vi "WriteBarcodeType.vi"(4 "error in (no error)":errorcluster, 5 "Value":T2, 6 "Container State":T3, 7 "Display State In":T1) -> (0 "error out":errorcluster, 3 "Display State Out":T1)   [LabVIEW 2013, in "BarCodes.lvlib" / "Barcode.xctl"]
uses:
  Barcode.xctl
  <vilib>/_xctls/Container State.ctl
  BarcodeType.ctl
  State.ctl
  <vilib>/_xctls/XControlSupport.lvlib
  BarCodes.lvlib
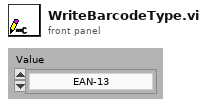
[diagram p1: front panel]
types:
  T1 = typedef "BarCodes.lvlib/Barcode.xctl/State.ctl" = cluster{"BarcodeType":T2, "Scale":u8, "Dark Color":u32, "Light Color":u32}
  T2 = typedef "BarCodes.lvlib/BarcodeType.ctl" = enum16{"EAN-13", "UPC", "Code 39 (3 of 9)", "Code 128"}
  T3 = typedef "XControlSupport.lvlib/Container State.ctl" = cluster{"Indicator?":bool, "Run Mode?":bool, " Refnum":refnum<vi>}
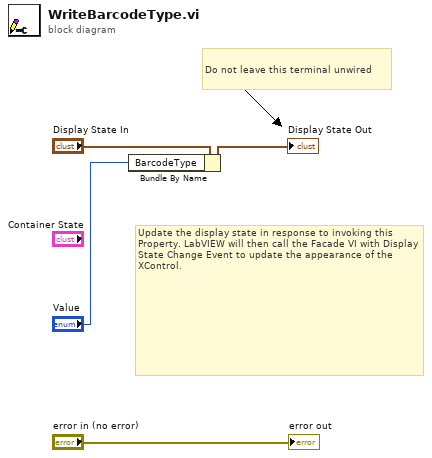
[diagram p0: block diagram]
diagram:
  # "Do not leave this terminal unwired"
  # "Update the display state in response to invoking this Property. LabVIEW will then call the Facade VI with Display State Change Event to update the appearance of the XControl."
  n1 = Bundle By Name(cluster="Display State In", "BarcodeType"="Value") -> (→"Display State Out":T1)
  "error out" <- "error in (no error)"
